vi "Test_Cleanup.vi"(8 "error in (no error)":errorcluster, 9 "Reset Supplies?":bool, 10 "Reset Refclk?":bool, 11 "Test Being Cleaned Up":string(combo)="Core/NB/DDR Test") -> (0 "error out":errorcluster)   [LabVIEW 2011]
doc: "This VI will cleanup the test that was just completed and return the PLL's back to the state they were in just after power up. This does NOT reset refclk or power supplies at this time.\n\nInputs:\n1. Test Being Cleaned UP: Specifies the type of test that was just run that will be cleaned up (Core/NB/DDR or HT).\n2. Reset Refclk?: If true resets the refclk to 200MHz\n3. Reset Supplies?: If true resets all of the power supplies to the power up voltage."
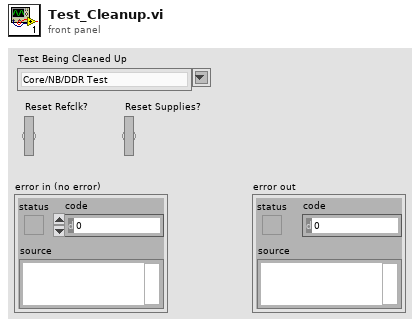
[diagram p1: front panel]
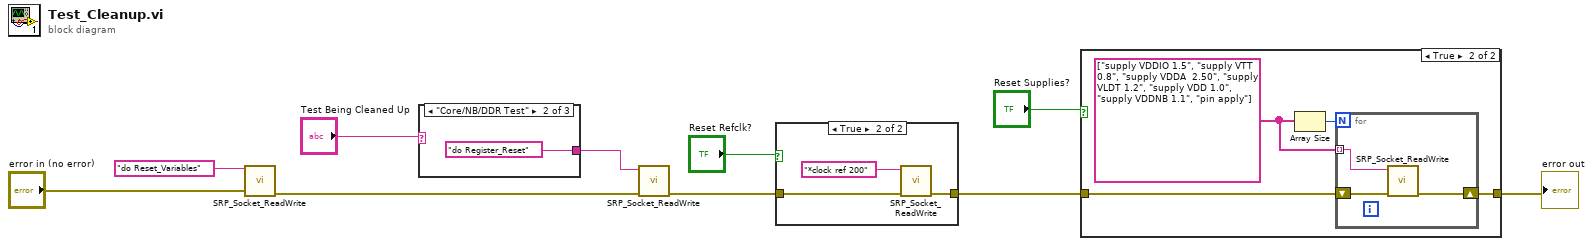
[diagram p0: block diagram]
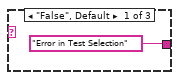
[diagram p4: hidden frame]
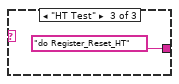
[diagram p5: hidden frame]
diagram:
  n1 = call "SRP_Socket_ReadWrite.vi"("error in (no error)"="error in (no error)", "Data In"="do Reset_Variables") -> ("error out"=w9:errorcluster)  [unwired: 7 in, 1 out]
  n2 = case shown="\"Core/NB/DDR Test\"" "Test Being Cleaned Up" {
    tunnel: ["Error in Test Selection" "do Register_Reset" "do Register_Reset_HT"] -> w6
    frame "False", Default {
    }
    frame "Core/NB/DDR Test" {
    }
    frame "HT Test" {
    }
  }
  n3 = call "SRP_Socket_ReadWrite.vi"("error in (no error)"=w9, "Data In"=w6) -> ("error out"=w4:errorcluster)  [unwired: 7 in, 1 out]
  n4 = case shown="True" "Reset Refclk?" {
    tunnel: w4 -> [w14 w15]
    tunnel: [w14 w16] -> w1
    frame False {
    }
    frame True {
      n5 = call "SRP_Socket_ReadWrite.vi"("error in (no error)"=w15, "Data In"="*clock ref 200") -> ("error out"=w16:errorcluster)  [unwired: 7 in, 1 out]
    }
  }
  n6 = case shown="True" "Reset Supplies?" {
    tunnel: [w18 w20] -> w2
    tunnel: w1 -> [w18 w19]
    frame False {
    }
    frame True {
      w22 = string[] ["supply VDDIO 1.5", "supply VTT 0.8", "supply VDDA  2.50", "supply VLDT 1.2", "supply VDD 1.0", "supply VDDNB 1.1", "pin apply"]
      n7 = Array Size(array=w22) -> (size(s)=w21:i32)
      n8 = for {
        N: w21 -> [_]
        tunnel: w22 -> [w23] mode=indexing
        shift-right: [w25] -> w20
        shift-left: w19 -> [w24]
        n9 = call "SRP_Socket_ReadWrite.vi"("error in (no error)"=w24, "Data In"=w23) -> ("error out"=w25:errorcluster)  [unwired: 7 in, 1 out]
      }
    }
  }
  "error out" <- w2
